vi "Test frame lookup.vi"() -> ()   [LabVIEW 2021]
uses:
  _Private/Data Classes/CAN Data Class/CAN Data.lvclass
  ENET_BS120x.lvclass
  <vilib>/xnet/xnet.llb/XNET Create Session (Conversion).vi
  <vilib>/xnet/xnet.llb/XNET Convert (Signal to Frame CAN).vi
  C:/Users/Public/Documents/Projects/7100-00109 SW BS1201 LV Driver/trunk/source/BS120x.lvclass
  C:/Users/Public/Documents/Projects/7100-00109 SW BS1201 LV Driver/trunk/source/ENET_BS120x/ENET_BS120x.lvclass
  C:/Users/Public/Documents/Projects/7100-00109 SW BS1201 LV Driver/trunk/source/_Private/Data Classes/Data Class/Data.lvclass
  C:/Users/Public/Documents/Projects/7100-00109 SW BS1201 LV Driver/trunk/source/_Private/Data Classes/CAN Data Class/CAN Data.lvclass
panel:
  out "Array":T1(array[cluster])
  out "data string 2":string
  out "data string":string
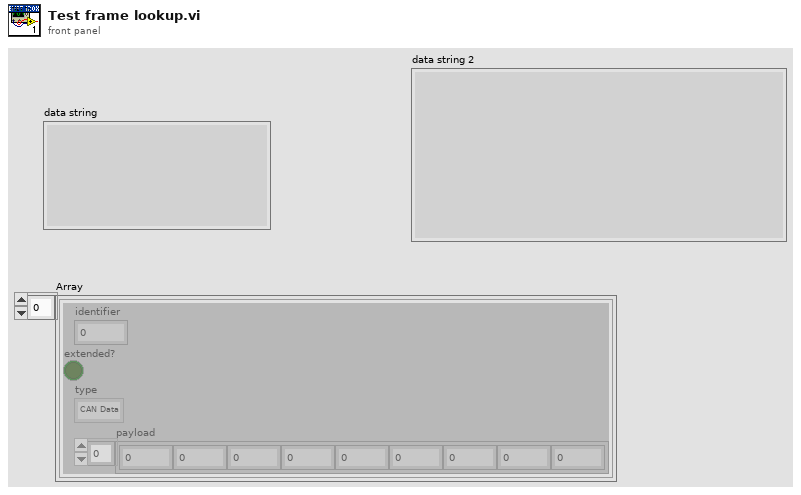
[diagram p1: front panel]
types:
  T1 = cluster{"identifier":u32, "extended?":bool, "type":enum8{"CAN Data", "CAN Remote"}, "payload":u8[]}[]
  T2 = cluster{"identifier":u32, "extended?":bool, "type":enum8{"CAN Data", "CAN Remote"}, "payload":u8[]}
  T3 = typedef "XNET Frame CAN.ctl" = cluster{"timestamp":timestamp, "payload":u8[], "identifier":u32, "type":T4, "extended?":bool, "echo?":bool}
  T4 = typedef "XNET Frame Type CAN.ctl" = u8
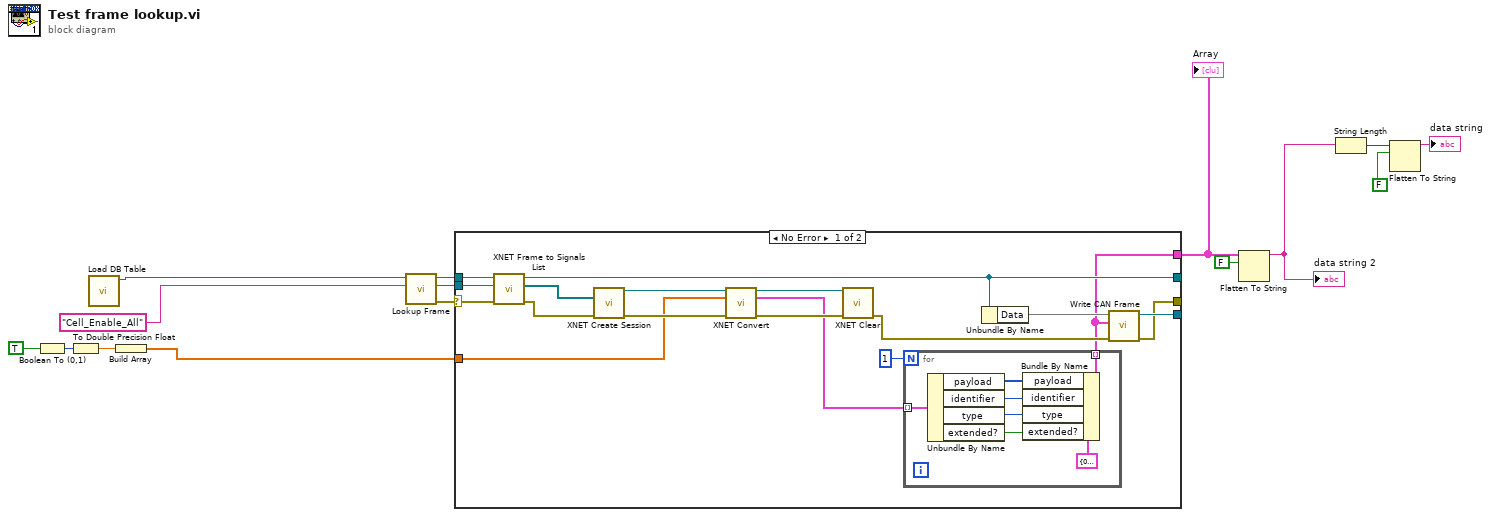
[diagram p0: block diagram]
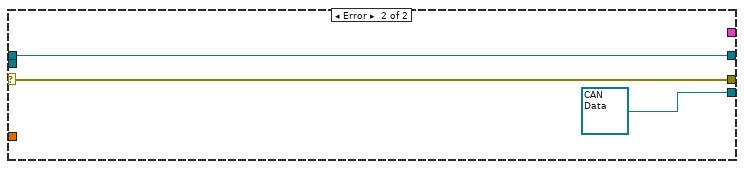
[diagram p2: hidden frame]
diagram:
  n1 = Boolean To (0,1)(Boolean=TRUE) -> (0, 1=w14:i16)
  n2 = To Double Precision Float(number=w14) -> (double precision float=w15:dbl)
  n3 = call-dynamic "Load DB Table.vi"() -> ("ENET out"=w9:refnum<class "ENET_BS120x.lvclass">)  [unwired: 10 in, 1 out]
  n4 = Build Array(w15) -> (w7:dbl[])
  n5 = call "Lookup Frame.vi"("Frame"="Cell_Enable_All", "Ethernet in"=w9) -> ("error out"=w11:errorcluster, "XNET Frame"=w10:refnum<k21>, "Ethernet out"=w12:refnum<class "ENET_BS120x.lvclass">)  [unwired: 7 in]
  n6 = case shown="No Error" w11 {
    selector: w11 -> [w24 w41]
    tunnel: [w25 w41] -> _
    tunnel: w7 -> [w31 _]
    tunnel: w12 -> [w20 w43]
    tunnel: [w18 w43] -> _
    tunnel: [w26 refnum<class "CAN Data.lvclass"> refnum ("CAN Data out")] -> _
    tunnel: w10 -> [w19 _]
    tunnel: [w16 _] -> w6
    frame No Error {
      # "CAN frame found"
      n7 = call-dynamic "XNET Frame to Signals List.vi"("error in (no error)"=w24, "XNET Frame"=w19, "BS1200 in"=w20) -> ("error out"=w23:errorcluster, "Sorted XNET Signals"=w21:refnum<k21>[], "BS1200 out"=w18:refnum<class "ENET_BS120x.lvclass">)  [unwired: 6 in]
      n8 = call-poly <vilib>:"XNET Create Session.vi"("signal list"=w21, "error in (no error)"=w23) -> ("session out"=w33:refnum<k21>, "error out"=w32:errorcluster)  [unwired: 12 out]
      n9 = call-poly <vilib>:"XNET Convert.vi"("session in"=w33, "signal data"=w31, "error in (no error)"=w32) -> ("session out"=w30:refnum<k21>, "frame data"=w28:T3[], "error out"=w29:errorcluster)  [unwired: 10 out]
      n10 = call <vilib>:"XNET Clear.vi"("session in"=w30, "error in (no error)"=w29) -> ("error out"=w22:errorcluster)  [unwired: 13 in]
      n11 = for {
        N: 1 -> [_]
        tunnel: w28 -> [w36] mode=indexing
        tunnel: [w35] -> w16 mode=indexing
        n12 = Unbundle By Name(w36) -> ("payload"=w37:u8[], "identifier"=w38:u32, "type"=w39:T4, "extended?"=w40:bool)
        n13 = Bundle By Name(cluster=T2 {"identifier"=0, "extended?"=FALSE, "type"=enum."CAN Data", "payload"=[0, 0, 0, 0, 0, 0, 0, 0]} ("CAN Frame"), "payload"=w37, "identifier"=w38, "type"=w39, "extended?"=w40) -> (w35:T2)
      }
      n14 = Unbundle By Name(w18) -> ("Data"=w17)
      n15 = call "Write CAN Frame.vi"("error in (no error)"=w22, "CAN Frame Array"=w16, "CAN Data in"=w17) -> ("error out"=w25:errorcluster, "CAN Data out"=w26:refnum<class "CAN Data.lvclass">)  [unwired: 7 in]
    }
    frame Error {
      # "CAN Frame not found"
    }
  }
  "Array" <- w6
  n16 = Flatten To String(anything=w6, prepend array or string size? (T)=FALSE) -> (data string=w2:string)  [unwired: 2 in, 2 out]
  "data string 2" <- w2
  n17 = String Length(string=w2) -> (length=w4:i32)
  n18 = Flatten To String(anything=w4, prepend array or string size? (T)=FALSE) -> (data string=→"data string":string)  [unwired: 2 in, 2 out]
